vi "MeasuredWalls_set.vi"(8 "error in (no error)":errorcluster, 10 "MeasuredWalls":T1(array[cluster])) -> (0 "error out":errorcluster)   [LabVIEW 2009, in "NetworkVarTarget.lvlib"]
uses:
  NetworkVarTarget.lvlib
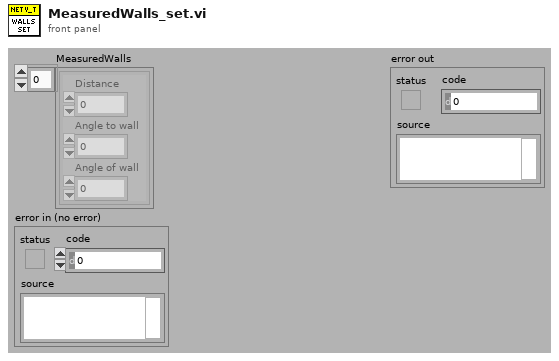
[diagram p1: front panel]
types:
  T1 = cluster{"Distance":dbl, "Angle to wall":dbl, "Angle of wall":dbl}[]
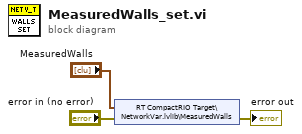
[diagram p0: block diagram]
diagram:
  n1 = shared-variable "RT CompactRIO Target\\NetworkVar.lvlib\\MeasuredWalls"("MeasuredWalls", error in="error in (no error)") -> (error out=→"error out":errorcluster)
